vi "Config Load Arm Globals.vi"(11 "refnum":T1) -> (3 "refnum 2":T1)   [LabVIEW 2012]
uses:
  <vilib>/Utility/config.llb/Config Data RefNum.ctl
  <vilib>/Utility/config.llb/Read Key (Double).vi
  <vilib>/Utility/config.llb/Read Key (I32).vi
  Arm Globals.vi
  <vilib>/Utility/config.llb/NI_LVConfig.lvlib
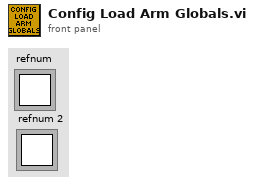
[diagram p1: front panel]
types:
  T1 = typedef "NI_LVConfig.lvlib/Config Data RefNum.ctl" = refnum<k1>
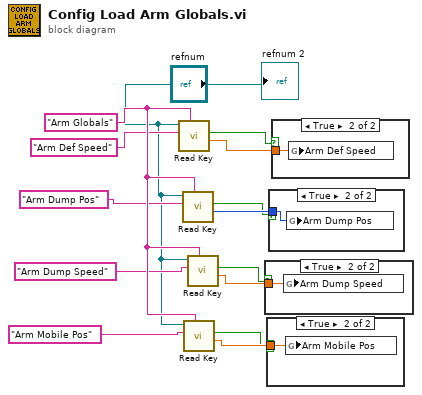
[diagram p0: block diagram]
diagram:
  w14 = "Arm Globals"
  n1 = call-poly <vilib>:"Read Key.vi"("section"=w14, "key"="Arm Def Speed", "refnum"="refnum") -> ("value"=w13:dbl, "found?"=w5:bool)  [unwired: 5 in, 2 out]
  n2 = call-poly <vilib>:"Read Key.vi"("section"=w14, "key"="Arm Dump Pos", "refnum"="refnum") -> ("value"=w8:i32, "found?"=w4:bool)  [unwired: 5 in, 2 out]
  n3 = call-poly <vilib>:"Read Key.vi"("section"=w14, "key"="Arm Mobile Pos", "refnum"="refnum") -> ("value"=w6:dbl, "found?"=w2:bool)  [unwired: 5 in, 2 out]
  n4 = call-poly <vilib>:"Read Key.vi"("section"=w14, "key"="Arm Dump Speed", "refnum"="refnum") -> ("value"=w7:dbl, "found?"=w3:bool)  [unwired: 5 in, 2 out]
  n5 = case shown="True" w3 {
    tunnel: w7 -> [_ w15]
    frame False {
    }
    frame True {
      n6 = global write "Arm Globals.vi" "Arm Dump Speed"(w15) -> ()
    }
  }
  n7 = case shown="True" w2 {
    tunnel: w6 -> [_ w16]
    frame False {
    }
    frame True {
      n8 = global write "Arm Globals.vi" "Arm Mobile Pos"(w16) -> ()
    }
  }
  n9 = case shown="True" w4 {
    tunnel: w8 -> [_ w17]
    frame False {
    }
    frame True {
      n10 = global write "Arm Globals.vi" "Arm Dump Pos"(w17) -> ()
    }
  }
  n11 = case shown="True" w5 {
    tunnel: w13 -> [_ w18]
    frame False {
    }
    frame True {
      n12 = global write "Arm Globals.vi" "Arm Def Speed"(w18) -> ()
    }
  }
  "refnum 2" <- "refnum"
